vi "VIQueryVersion.vi"(8 "Error In":errorcluster, 11 "VI Path":string) -> (0 "Error Out":errorcluster, 3 "Version":string)   [LabVIEW 2013]
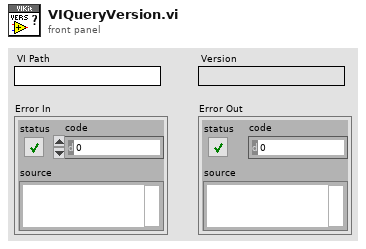
[diagram p1: front panel]
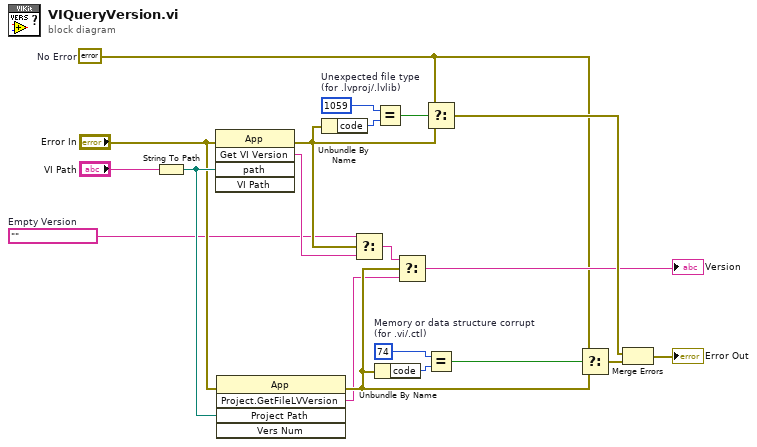
[diagram p0: block diagram]
diagram:
  w2 = errorcluster {"status"=FALSE, "code"=0, "source"=""}  # No Error
  w1 = ""  # Empty Version
  w12 = 74  # Memory or data structure corrupt (for .vi/.ctl)
  w16 = 1059  # Unexpected file type (for .lvproj/.lvlib)
  n1 = String To Path(string="VI Path") -> (path=w19:path)
  n2 = invoke class="App" method="Get VI Version"(error in="Error In", "path"=w19) -> (error out=w14:errorcluster, "GetVIVers"=w20:string)  [unwired: 3 in, 3 out]
  n3 = invoke class="App" method="Project.GetFileLVVersion"(error in="Error In", "Project Path"=w19) -> (error out=w10:errorcluster, "Project.GetFileLVVersion"=w7:string)  [unwired: 3 in, 3 out]
  n4 = Unbundle By Name(w14) -> ("code"=w15:i32)
  n5 = Select(t=w1, s=w14, f=w20) -> (s? t:f=w18:string)
  n6 = Equal?(x=w16, y=w15) -> (x = y?=w17:bool)
  n7 = Unbundle By Name(w10) -> ("code"=w13:i32)
  n8 = Select(t=w18, s=w10, f=w7) -> (s? t:f=→"Version":string)
  n9 = Select(t=w2, s=w17, f=w14) -> (s? t:f=w9:errorcluster)
  n10 = Equal?(x=w12, y=w13) -> (x = y?=w11:bool)
  n11 = Select(t=w2, s=w11, f=w10) -> (s? t:f=w8:errorcluster)
  n12 = Merge Errors(w9, w8) -> (→"Error Out":errorcluster)
